vi "Write Config.vi"(8 "error in (no error)":errorcluster, 9 "Re-Init?":bool, 10 "ICM File In":path, 11 "Modbus in":refnum<class "Modbus.lvclass">) -> (0 "error out":errorcluster, 3 "Modbus out":refnum<class "Modbus.lvclass">)   [LabVIEW 2024, in "Modbus.lvclass"]
doc: "Modbus.lvclass:Write Config.vi\n\nThis VI writes the Modbus configuration to the configuration file.\n\nInstrument Communication Module Version 1.0\nJanuary, 2018 Original Code Consulting David Thomson\n www.originalcode.com"
uses:
  Modbus.lvclass
  Modbus.lvclass/Modbus.ctl
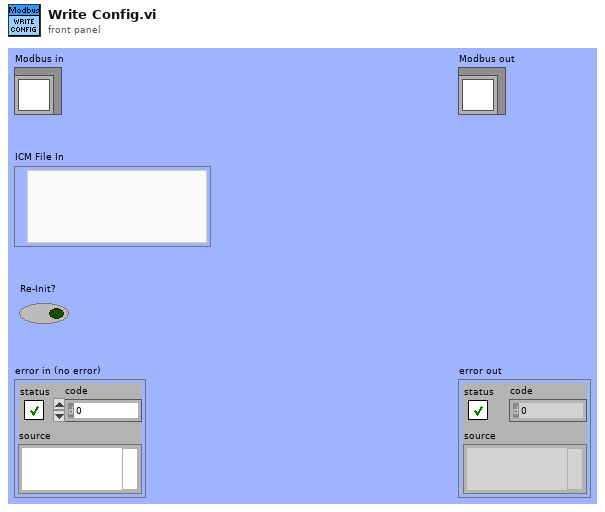
[diagram p1: front panel]
types:
  T1 = typedef "Modbus Config.ctl" = cluster{"Port":u16, "Modbus Server Name":string, "Serial/Ethernet":bool, "Baud Rate":u32, "Serial Type":enum16{"RTU", "ASCII"}, "Unit ID":u8, "Parity":u16, "Input Channels":cluster{"Data Type":T2, "Address":u16}[], "Swap Words?":bool}
  T2 = typedef "ICM Modbus Data Type.ctl" = enum16{"Boolean", "U16 (unsigned 16bit Int)", "I16 (signed 16bit Int)", "U32 (unsigned 32bit Int)", "I32 (signed 32bit Int)", "Real (Single 32bit)"}
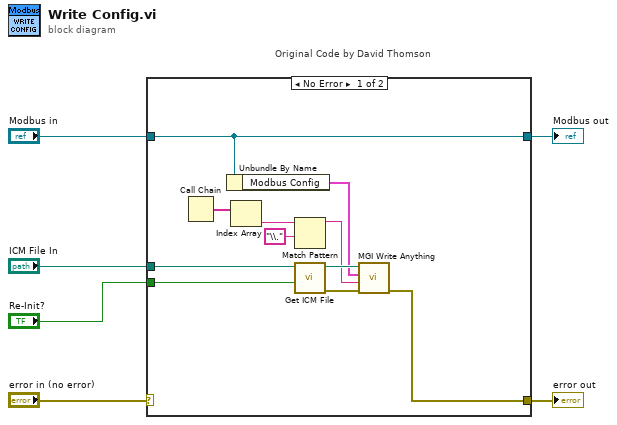
[diagram p0: block diagram]
diagram:
  n1 = case "Original Code by David Thomson" shown="No Error" "error in (no error)" {
    selector: "error in (no error)" -> [_ w19]
    tunnel: [w9 w19] -> w4
    tunnel: [w14 w18] -> w3
    tunnel: "Modbus in" -> [w14 w18]
    tunnel: "ICM File In" -> [w8 _]
    tunnel: "Re-Init?" -> [w7 _]
    frame No Error {
      n2 = Call Chain() -> (call chain=w16:string[])
      n3 = Unbundle By Name(w14) -> ("Modbus Config"=w10:T1)
      n4 = Index Array(array=w16) -> (element=w15:string)  [unwired: 1 in]
      n5 = Match Pattern(string=w15, regular expression="\\.") -> (before substring=w11:string)  [unwired: 1 in, 3 out]
      n6 = call "Get ICM File.vi"("Re-Init?"=w7, "ICM File In"=w8) -> ("error out"=w13:errorcluster, "ICM File"=w12:path)  [unwired: 8 in]
      n7 = call <userlib>:"MGI Write Anything.vi"("Error In"=w13, "Section Name (Name of \"Anything\")"=w11, "Anything"=w10, "Path (dialog)"=w12) -> ("Error Out"=w9:errorcluster)  [unwired: 5 in, 2 out]
    }
    frame Error {
    }
  }
  "error out" <- w4
  "Modbus out" <- w3
